vi "Agilent 546XX Series Acq Digital Wfm Edge Triggered.vi"() -> ()   [LabVIEW 2014]
doc: "DESCRIPTION:\nThis VI shows how to configure the ag546xx for digital channel waveform acquisition. It uses edge triggering to trigger the acquisition. \n\nINSTRUCTIONS:\n1. Pass a valid instrument VISA session into this VI.\n2. Enter Threshold and User Value if needed.\n3. Enter the acquisition start time and desired time per record.\n4. Enter the trigger level for the edge trigger.\n5. Run the VI.\n6. The acquired waveform will be displayed in the graph.\n\nNOTES:\nNotice the order of the ag546xx component VIs in the block diagram. The first VI in this sequence accepts a valid instrument VISA session which provides a dup VISA session to the instrument driver. The instrument session is generated by the ag546xx Initialize.vi. The last VI in the sequence passes the VISA session out. \n\nThis VI sets the following controls on the block diagram:\n Input Impedance: 100E+3 Ohms\n 200 ns Trigger Holdoff\n Edge trigger is DC coupled with a positive slope.\nTo change these values, modify the associated block diagram constants."
uses:
  <vilib>/Waveform/DWDTOps.llb/DWDT Boolean Array to Digital.vi
  <instrlib>/Agilent 546XX Series/Agilent 546XX Series.lvlib
panel:
  in  "Serial Configuration":cluster{"Baud Rate":u32, "Flow Control":u16}={"Baud Rate"=0, "Flow Control"=4} {"Flow Control" items=["None", "XON/XOFF", "RTS/CTS", "XON/XOFF & RTS/CTS", "DTR/DSR", "XON/XOFF & DTR/DSR"]; "Baud Rate" items=["9600", "19200", "38400", "57600"]}
  out "Digital Waveform Graph":digitalwaveform(graph)
  in  "Read Digital Group (\"POD1&2\")":string(combo)="BOTH"
  in  "user value (0.0 V)":dbl caption="User Value (0.0 V)" format="%^.2e"
  in  "Threshold (TTL)":string(combo)="TTL"
  in  "Configure Channel (\"D0\")":string(combo)="DIG0"
  in  "acquisition start time (0.0 sec)":dbl caption="Acquisition Start Time (0.0 sec)" format="%^.2e"
  in  "time per record (20.0E-3 sec)":dbl=0.002 caption="Time Per Record (2.0E-3 sec)" format="%^.2e"
  in  "minimum record length (1000)":i32=1000 caption="Min Record Length (1000 samples)"
  in  "trigger level (0.0 volts)":dbl=1.4 caption="Trigger Level (1.4 volts)" format="%^.2e"
  in  "VISA Resource Name":refnum<visa-resource-name> caption="VISA session"
  # "© 2003, National Instruments, Corporation.  All Rights Reserved."
  # "For instructions,\nselect Show Context Help\nfrom the Help menu."
  # "Time is relative to the first point and not the actual start time before / after trigger"
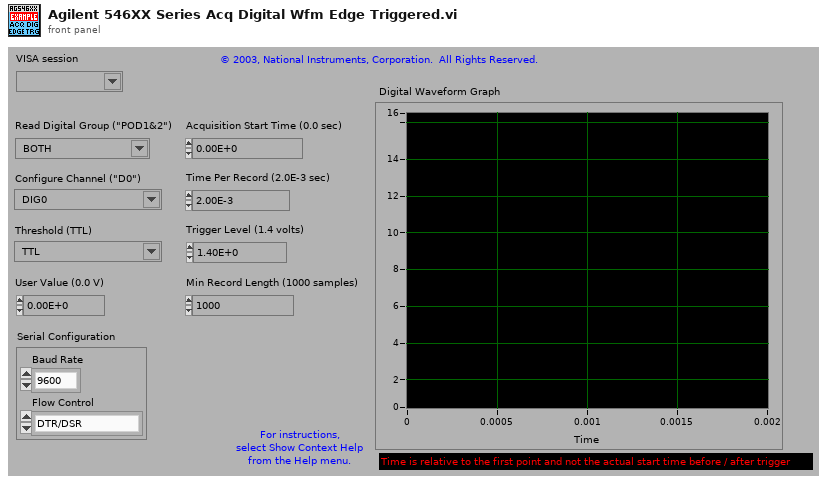
[diagram p1: front panel]
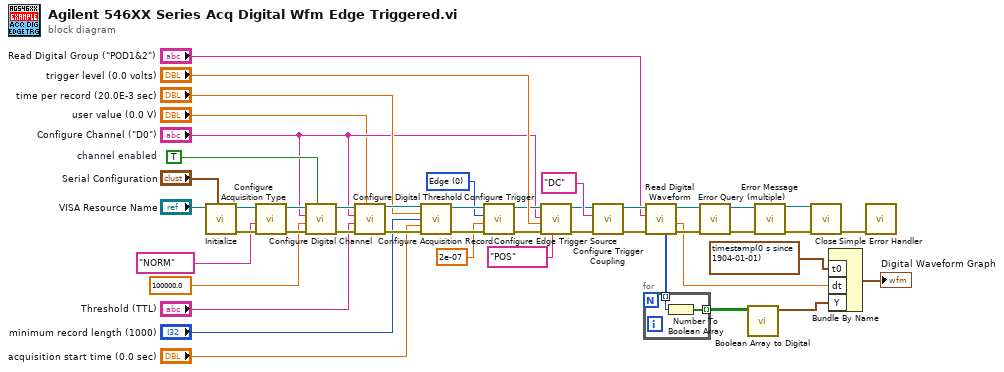
[diagram p0: block diagram]
diagram:
  w30 = 0 items=["Edge", "Glitch", "TV", "AC Line", "Pattern", "Duration", "IIC", "Sequence"] ("Trigger Type (Edge)")
  w21 = TRUE  # channel enabled
  n1 = call <instrlib>:"Initialize.vi"("Serial Configuration"="Serial Configuration", "VISA Resource Name"="VISA Resource Name") -> ("error out"=w45:errorcluster, "VISA Resource Name Out"=w8:refnum<visa-resource-name>)  [unwired: 8 in]
  n2 = call <instrlib>:"Configure Acquisition Type.vi"("error in (no error)"=w45, "Acquisition Type (Sample)"="NORM", "VISA Resource Name"=w8) -> ("error out"=w44:errorcluster, "VISA Resource Name Out"=w42:refnum<visa-resource-name>)  [unwired: 7 in]
  n3 = call <instrlib>:"Configure Digital Channel.vi"("channel enabled (True)"=w21, "error in (no error)"=w44, "input impedance (100.0E+3 ohms)"=100000.0, "Digital Channel (\"D0\")"="Configure Channel (\"D0\")", "VISA Resource Name"=w42) -> ("error out"=w43:errorcluster, "VISA Resource Name Out"=w32:refnum<visa-resource-name>)  [unwired: 5 in]
  n4 = call <instrlib>:"Configure Digital Threshold.vi"("user value (0.0 V)"="user value (0.0 V)", "error in (no error)"=w43, "Threshold (TTL)"="Threshold (TTL)", "Digital Channel (\"D0\")"="Configure Channel (\"D0\")", "VISA Resource Name"=w32) -> ("error out"=w38:errorcluster, "VISA Resource Name Out"=w40:refnum<visa-resource-name>)  [unwired: 5 in]
  n5 = call <instrlib>:"Configure Acquisition Record.vi"("VISA Resource Name"=w40, "Time Per Record (1.0e-3 s)"="time per record (20.0E-3 sec)", "Minimum Record Length (2000)"="minimum record length (1000)", "Acquisition Start Time (0.0 s)"="acquisition start time (0.0 sec)", "error in (no error)"=w38) -> ("VISA Resource Name Out"=w34:refnum<visa-resource-name>, "error out"=w35:errorcluster)  [unwired: 9 in]
  n6 = call <instrlib>:"Configure Trigger.vi"("error in (no error)"=w35, "trigger holdoff (60.0E-9 s)"=2e-07, "Trigger Type (Edge)"=w30, "VISA Resource Name"=w34) -> ("error out"=w26:errorcluster, "VISA Resource Name Out"=w27:refnum<visa-resource-name>)  [unwired: 6 in]
  n7 = call <instrlib>:"Configure Edge Trigger Source.vi"("Trigger Slope (Positive)"="POS", "error in (no error)"=w26, "Trigger Level (0.0 V)"="trigger level (0.0 volts)", "Trigger Source (Channel 1)"="Configure Channel (\"D0\")", "VISA Resource Name"=w27) -> ("error out"=w24:errorcluster, "VISA Resource Name Out"=w25:refnum<visa-resource-name>)  [unwired: 5 in]
  n8 = call <instrlib>:"Configure Trigger Coupling.vi"("error in (no error)"=w24, "Trigger Coupling (DC)"="DC", "VISA Resource Name"=w25) -> ("error out"=w22:errorcluster, "VISA Resource Name Out"=w23:refnum<visa-resource-name>)  [unwired: 7 in]
  n9 = call <instrlib>:"Read Digital Waveform.vi"("error in (no error)"=w22, "Channel Name (\"POD1\")"="Read Digital Group (\"POD1&2\")", "VISA Resource Name"=w23) -> ("error out"=w46:errorcluster, "x increment"=w14:dbl, "VISA Resource Name Out"=w7:refnum<visa-resource-name>, "waveform array"=w11:u16[])  [unwired: 3 in, 2 out]
  n10 = for {
    tunnel: [w48] -> w15 mode=indexing
    tunnel: w11 -> [w47] mode=indexing
    n11 = Number To Boolean Array(number=w47) -> (Boolean array=w48:bool[])
  }
  n12 = call <instrlib>:"Error Query (multiple).vi"("error in (no error)"=w46, "VISA Resource Name"=w7) -> ("error out"=w4:errorcluster, "VISA Resource Name Out"=w6:refnum<visa-resource-name>)  [unwired: 6 in, 2 out]
  n13 = call-poly <vilib>:"Boolean Array to Digital.vi"("boolean array"=w15) -> ("digital waveform"=w13:digitalwaveform)  [unwired: 9 in, 1 out]
  n14 = call <instrlib>:"Error Message.vi"("VISA Resource Name"=w6, "error in (no error)"=w4) -> ("VISA Resource Name Out"=w5:refnum<visa-resource-name>, "error out"=w3:errorcluster)  [unwired: 9 in, 3 out]
  n15 = call <instrlib>:"Close.vi"("error in (no error)"=w3, "VISA Resource Name"=w5) -> ("error out"=w2:errorcluster)  [unwired: 9 in]
  n16 = Bundle By Name("t0"=timestamp(0 s since 1904-01-01), "dt"=w14, "Y"=w13) -> (→"Digital Waveform Graph":digitalwaveform)  [unwired: 1 in]
  n17 = call <vilib>:"Simple Error Handler.vi"("error in (no error)"=w2) -> ()  [unwired: 4 in, 5 out]
